vi "TDMS_export_tool.vi"() -> ()   [LabVIEW 2018]
doc: "Tool for exporting TDMS files into CSV format."
uses:
  <vilib>/Utility/miscctls.llb/LVPointTypeDef.ctl
  <vilib>/Platform/TimedLoop/XDataNode/timing_clust.ctl
  <vilib>/Platform/TimedLoop/XDataNode/nitl_modes.ctl
  <vilib>/Platform/TimedLoop/XDataNode/wakeup.ctl
  <vilib>/Utility/sysdir.llb/System Directory Type.ctl
  <vilib>/Platform/TimedLoop/scheduler/LVUserAPI/_suppVIs/Create_1kHz_TSource.vi
  <vilib>/Utility/file.llb/Write Delimited Spreadsheet (string).vi
  <vilib>/platform/TimedLoop/XDataNode/XDataNode.xnode
  <vilib>/Platform/TimedLoop/XDataNode/XDNodeRunTimeDep.lvlib
panel:
  out "error out":errorcluster
  out "Files converted":u32
  out "Settings":bool[](array[boolean])
  out "Data":bool[](array[boolean])
  out "Errors array":string[](array[string])
  in  "Convert":bool
  out "Files to convert":u32
  out "Filelist":path[](array[path])
  in  "Open Folder":bool caption="Open File"
  in  "Stop":bool
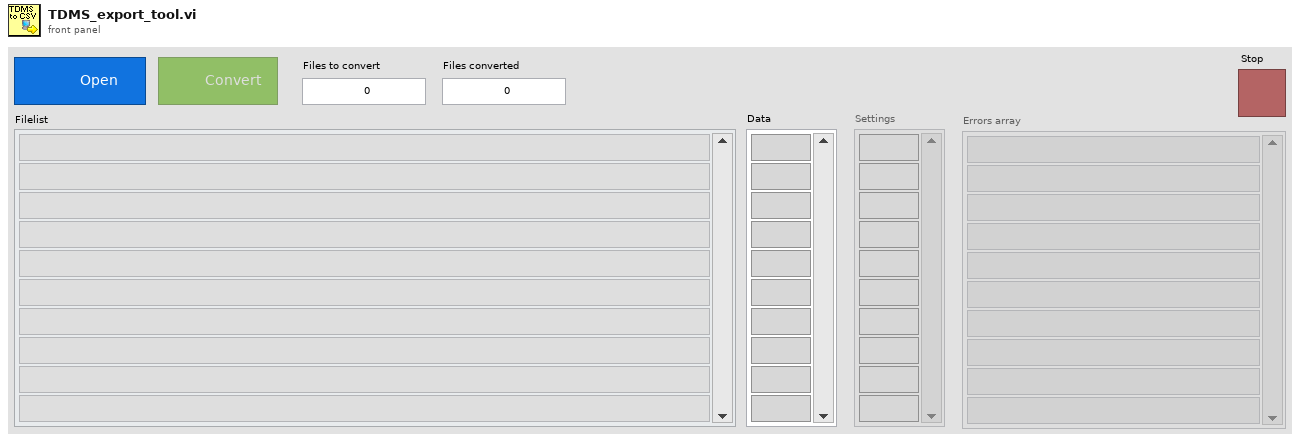
[diagram p1: front panel]
types:
  T1 = enum8{"Enabled", "Disabled", "Disabled and Grayed Out"}
  T2 = typedef "LVPointTypeDef.ctl" = cluster{"Horizontal":i16, "Vertical":i16}
  T3 = typedef "XDNodeRunTimeDep.lvlib/timing_clust.ctl" = cluster{"Expected End [f-1]":u64, "Actual End [f-1]":u64, "Finished Late? [f-1]":bool, "Expected End [i-1]":u64, "Actual End [i-1]":u64, "Finished Late? [i-1]":bool, "Expected Start [i]":u64, "Actual Start [i]":u64, "Expected Start [f]":u64, "Actual Start [f]":u64, "Source Name":string, "Structure Name":string, "Period":i64, "Deadline":i64, "Offset":i64, "Start":i64, "Priority":i32, "Timeout":i32, "Mode":T4, "Wakeup Reason":T5, "Error":errorcluster, "Source Type":string, "Secondary Source Type":string, "Global End Time":u64, "Global Start Time":u64, "Frame Duration":u64, "Iteration Duration":u64, "Assigned CPU":i32, "I/O Scan Engine Mode":u32}
  T4 = typedef "XDNodeRunTimeDep.lvlib/nitl_modes.ctl" = enum32{"No Change", "Process missed periods, maintain original phase", "Discard missed periods, maintain original phase", "Process missed periods, ignore original phase", "Discard missed periods, ignore original phase"}
  T5 = typedef "XDNodeRunTimeDep.lvlib/wakeup.ctl" = enum32{"Normal", "Aborted", "Asynchronous wakeup", "Timing source error", "Timed loop error", "Timeout"}
  T6 = enum32{"invalid app kind", "Development System", "Run Time System", "Student Edition", "Embedded LabVIEW", "Evaluation", "Custom"}
  T7 = typedef "System Directory Type.ctl" = i32
  T8 = cluster{"Raw coordinates data":dbl[][], "Absolute timestamp":string[], "Relative timestamp":string[], "Coordinates and speed":dbl[][], "Current zone and TTLs":u8[][], "Zones preference":string[], "Frame OK":u8[], "Stimulus presets array":cluster{"Event type":u16, "Time, s":sgl, "Stimulus, s":sgl, "Set/Clear":bool, "TTL out":u16, "Stim. has been set":bool}[], "Acquisition settings cluster out":cluster{"Researcher name":string, "N segments MIDFIELD":u8, "N segments BORDER":u8, "Radius, mm CENTER":u16, "Radius, mm MIDFIELD":u16, "Starting angle MIDFIELD":i16, "Starting angle BORDER":i16, "Cage diameter, mm":u16, "Bridge swap":bool, "Bridge V. offset":sgl, "Twisted neck":bool, "Offset H.":sgl, "Name prefix":string, "Stop at":dbl, "\"Stop at\" enabled":bool, "Settings loaded OK":bool}}
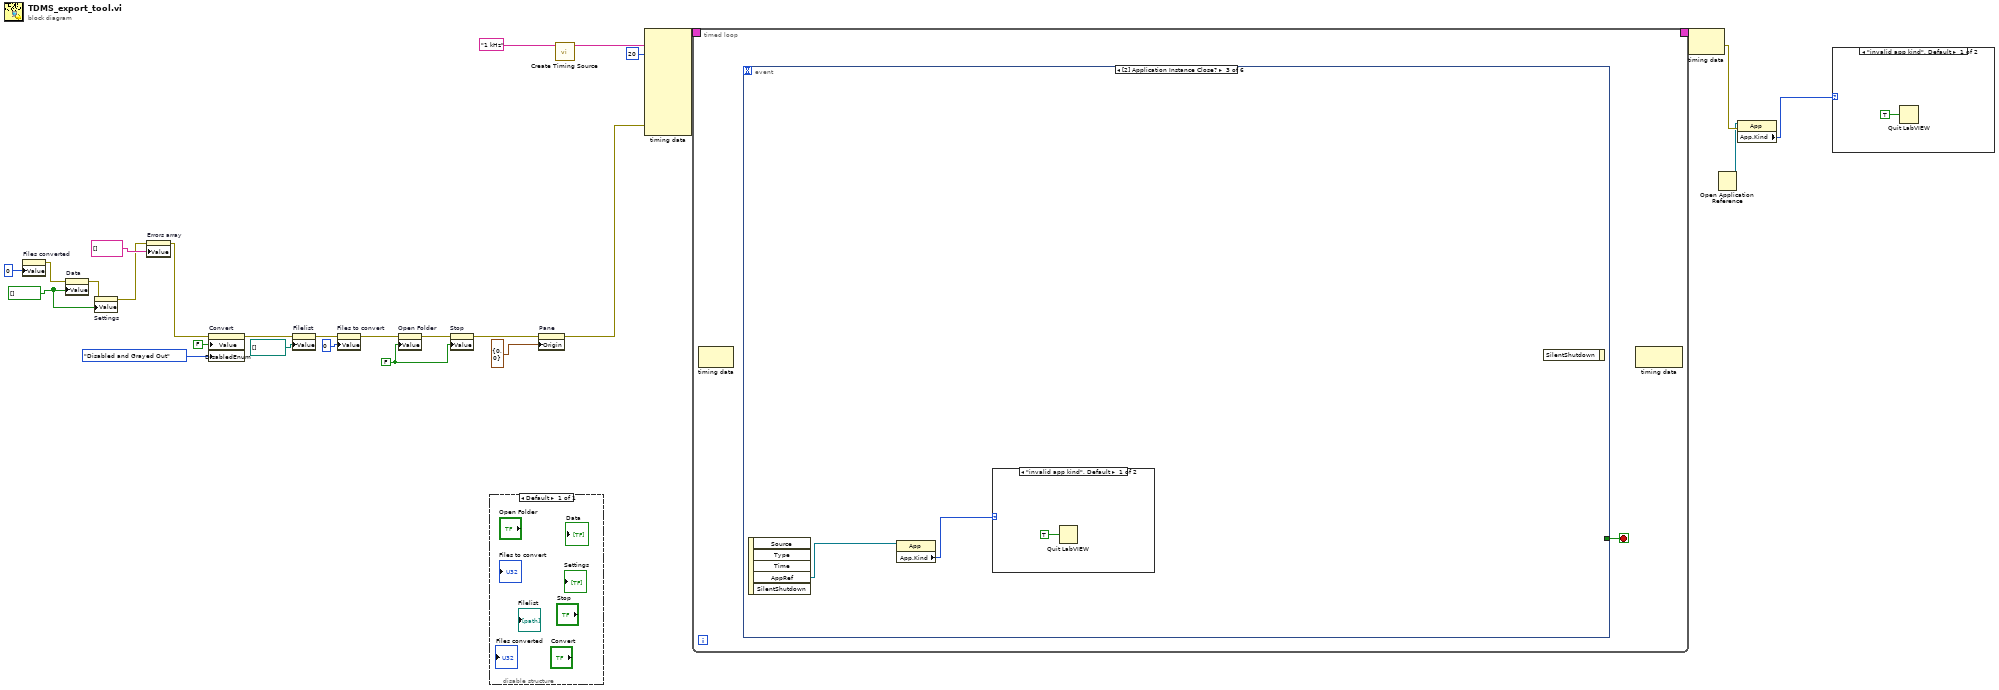
[diagram p0: block diagram]
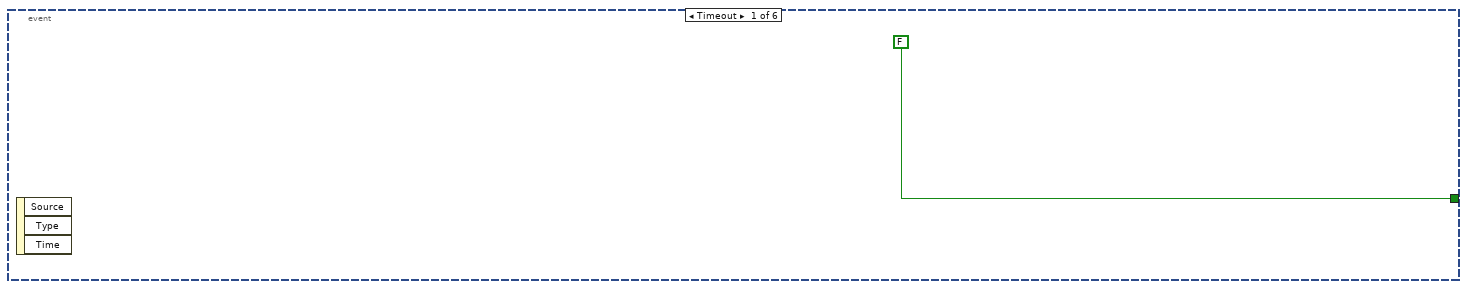
[diagram p3: hidden frame]
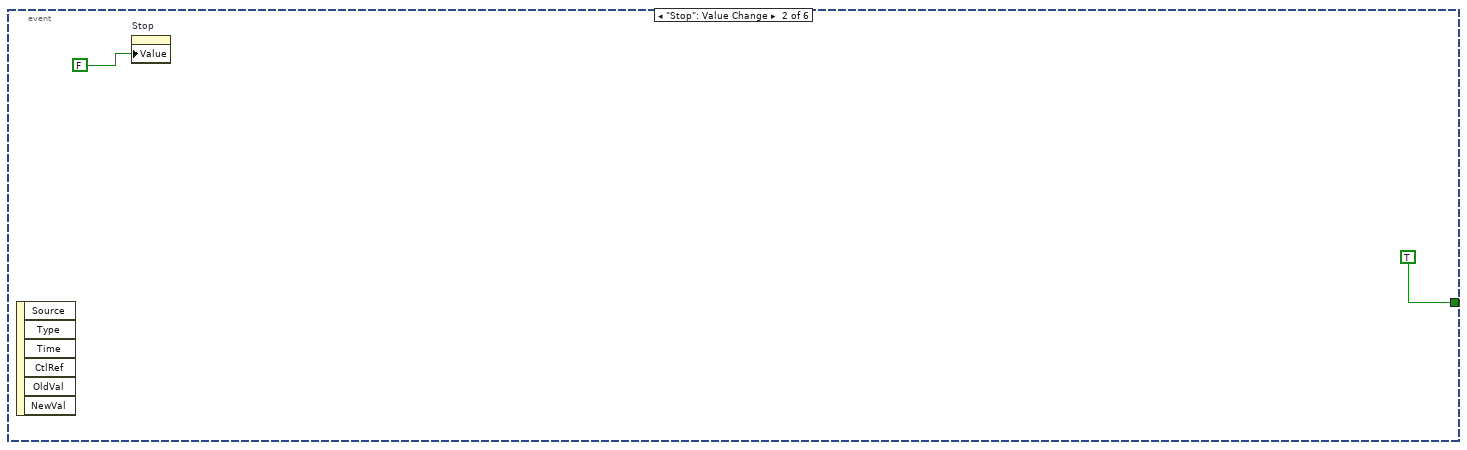
[diagram p4: hidden frame]
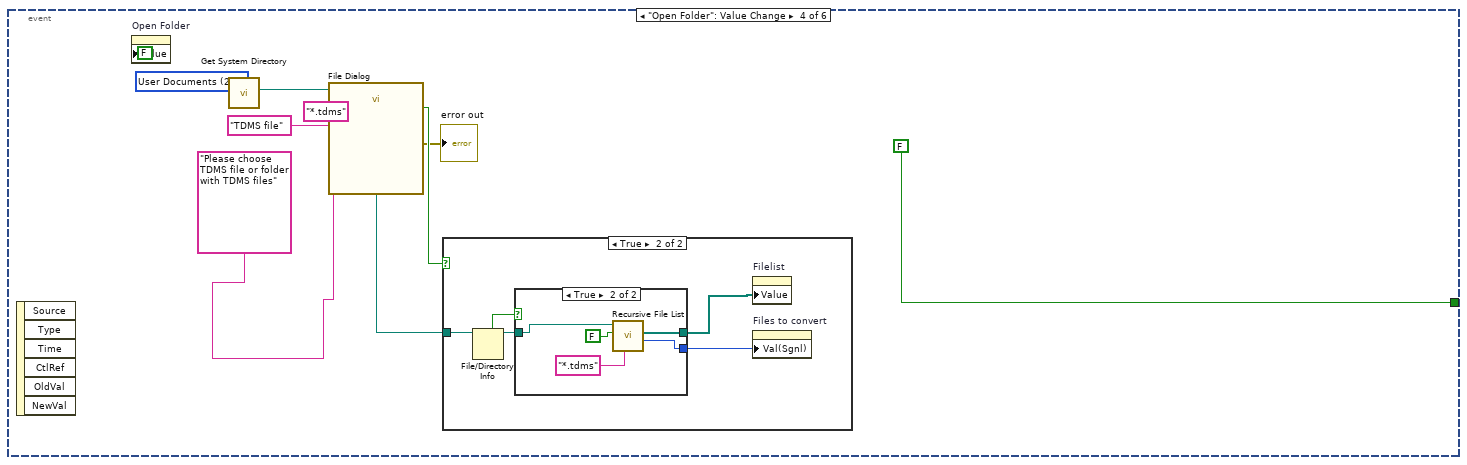
[diagram p6: hidden frame]
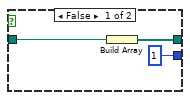
[diagram p8: hidden frame]
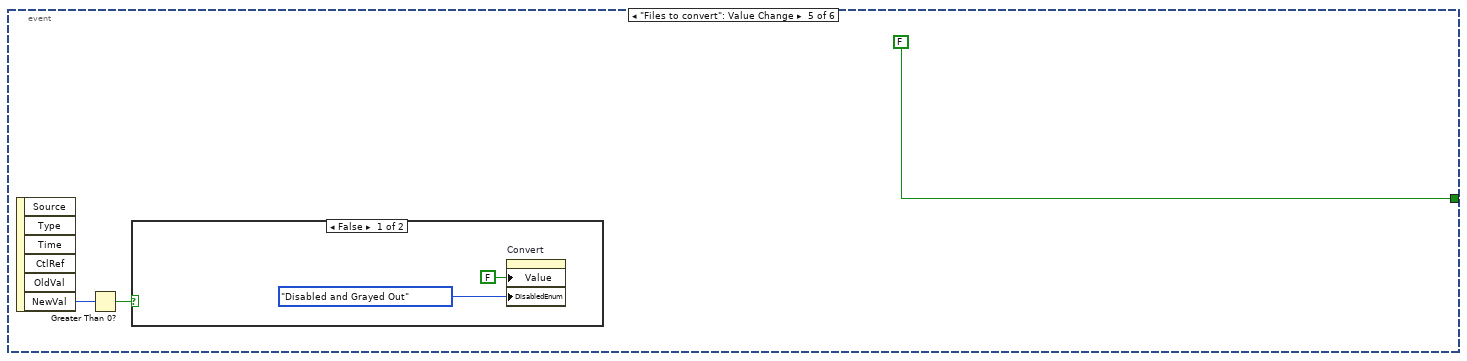
[diagram p9: hidden frame]
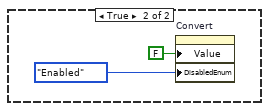
[diagram p10: hidden frame]
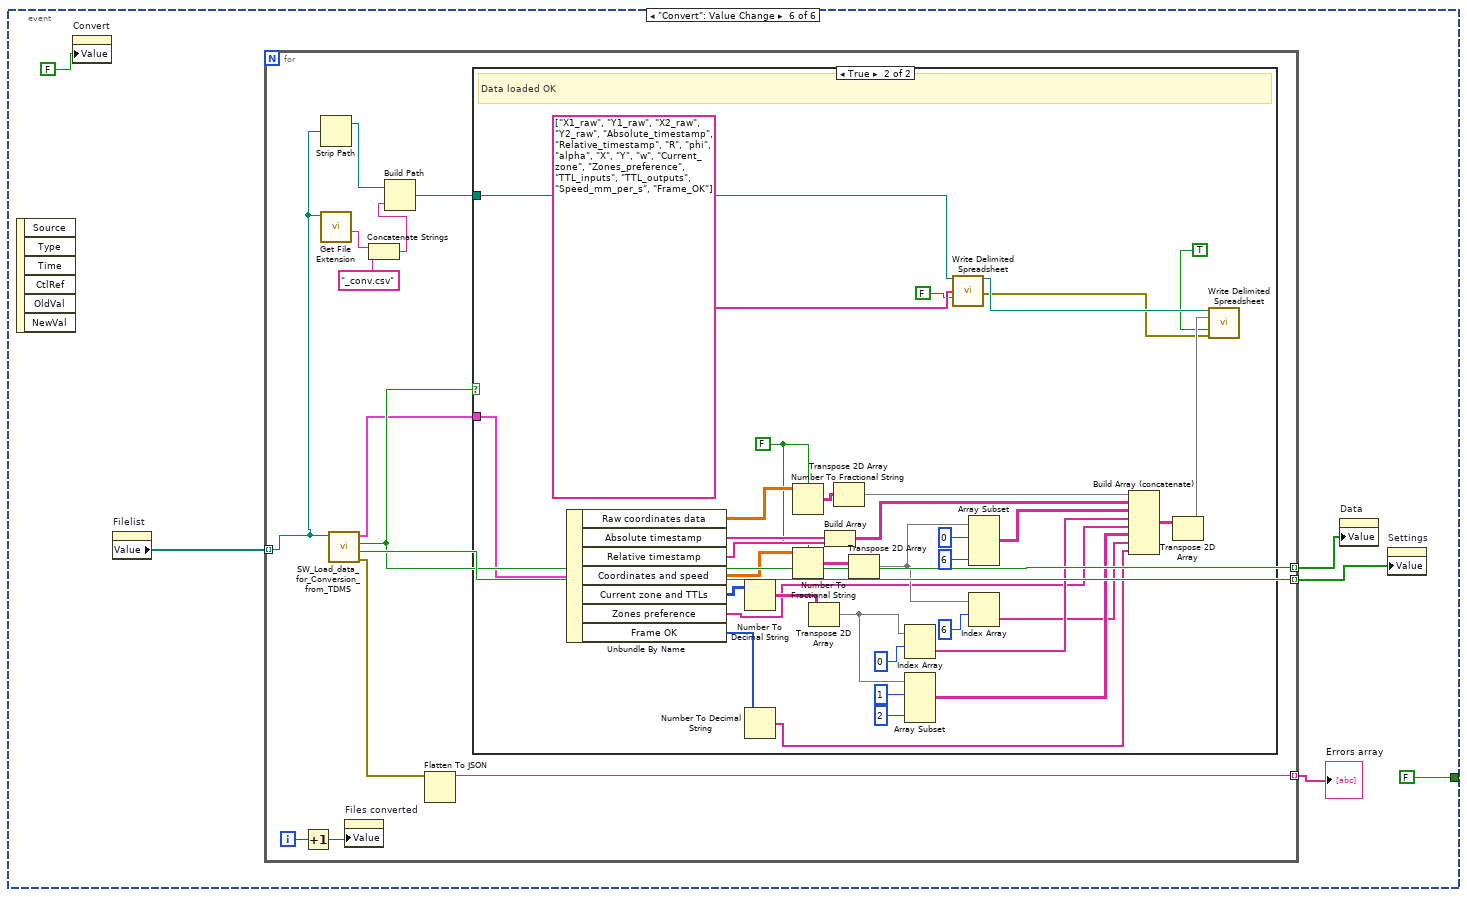
[diagram p11: hidden frame]
diagram:
  w8 = bool[] [] ("Array")
  w18 = FALSE ("Stop")
  n1 = property on="Files converted" class="DigNum (strict)"("Value"=u32 0 ("Files to converted")) -> (error out=w5:errorcluster)  [unwired: 2 in, 1 out]
  n2 = property on="Data" class="Arr"(error in=w5, "Value"=w8) -> (error out=w7:errorcluster)  [unwired: 1 in, 1 out]
  n3 = property on="Settings" class="Arr"(error in=w7, "Value"=w8) -> (error out=w6:errorcluster)  [unwired: 1 in, 1 out]
  n4 = property on="Errors array" class="Arr (strict)"(error in=w6, "Value"=string[] []) -> (error out=w10:errorcluster)  [unwired: 1 in, 1 out]
  n5 = property on="Convert" class="Bool (strict)"(error in=w10, "Value"=FALSE ("Convert"), "DisabledEnum"=T1."Disabled and Grayed Out" ("Disabled")) -> (error out=w13:errorcluster)  [unwired: 1 in, 1 out]
  n6 = property on="Filelist" class="Arr (strict)"(error in=w13, "Value"=path[] [] ("Files to process")) -> (error out=w14:errorcluster)  [unwired: 1 in, 1 out]
  n7 = property on="Files to convert" class="DigNum (strict)"(error in=w14, "Value"=u32 0 ("Number of files")) -> (error out=w17:errorcluster)  [unwired: 1 in, 1 out]
  n8 = property on="Open Folder" class="Bool (strict)"(error in=w17, "Value"=w18) -> (error out=w19:errorcluster)  [unwired: 1 in, 1 out]
  n9 = property on="Stop" class="Bool (strict)"(error in=w19, "Value"=w18) -> (error out=w20:errorcluster)  [unwired: 1 in, 1 out]
  n10 = disable-structure shown="Default" {
    frame Enabled {
    }
  }
  n11 = property on="Pane" class="Pane"(error in=w20, "Origin"=T2 {"Horizontal"=0, "Vertical"=0}) -> (error out=w21:errorcluster)  [unwired: 1 in, 1 out]
  n12 = call-poly <vilib>:"Create Timing Source.vi"("name (in)"="1 kHz") -> ("name (out)"=w24:string)  [unwired: 9 in, 1 out]
  n13 = node-c288(w24, i64 20 ("Period"), w21) -> (w27:T3)  [unwired: 7 in]
  n14 = timed-loop {
    timing: w27 -> [_]
    timing-out: [_] -> w26
    stop <- w28 stop-if-true
    n15 = node-c288() -> ()  [unwired: 1 in, 1 out]
    n16 = event shown="[2] Application Instance Close?" {
      selector: _ -> [_ _ _ _ _ _]
      dyn-events: _ -> [_ _ _ _ _ _]
      timeout: _ -> [_ _ _ _ _ _]
      tunnel: [FALSE TRUE _ FALSE FALSE FALSE] -> w28
      event Timeout {
        n17 = event-data() -> ()  [unwired: 1 in, 3 out]
      }
      event "Stop": Value Change {
        n18 = event-data() -> ()  [unwired: 1 in, 6 out]
        n19 = property on="Stop" class="Bool (strict)"("Value"=FALSE ("Stop")) -> ()  [unwired: 2 in, 2 out]
      }
      event Application Instance Close? {
        n20 = event-data() -> ("AppRef"=w33:refnum<vi>)  [unwired: 1 in, 4 out]
        n21 = property class="App"(reference=w33) -> ("App.Kind"=w32:T6)  [unwired: 1 in, 2 out]
        n22 = case shown="\"invalid app kind\", Default" w32 {
          frame "invalid app kind", Default {
            n23 = Quit LabVIEW(quit? (T)=TRUE) -> ()
          }
          frame "Development System" {
          }
        }
        n24 = event-data() -> ()  [unwired: 2 in, 1 out]
      }
      event "Open Folder": Value Change {
        w40 = T7 2 items=["User Home"=0, "User Desktop"=1, "User Documents"=2, "User Application Data"=3, "User Preferences"=4, "User Temporary"=5, "Public Documents"=6, "Public Application Data"=7, "Public Preferences"=8, "Public Cache"=13, "System Core Libraries"=9, "System Installed Libraries"=10, "Application Files"=11, "Boot Volume Root"=12] ("system directory type")
        n25 = event-data() -> ()  [unwired: 1 in, 6 out]
        n26 = property on="Open Folder" class="Bool (strict)"("Value"=FALSE ("Open Folder")) -> ()  [unwired: 2 in, 2 out]
        n27 = call <vilib>:"Get System Directory.vi"("system directory type"=w40) -> ("system directory"=w39:path)  [unwired: 10 in]
        n28 = call "File Dialog"("start path"=w39, "prompt"="Please choose TDMS file or folder with TDMS files", "pattern (all files)"="*.tdms", "pattern label"="TDMS file") -> ("selected path"=w36:path, "exists"=w37:bool, "error out"=→"error out":errorcluster)  [unwired: 8 in, 1 out]
        n29 = case shown="True" w37 {
          tunnel: w36 -> [_ w49]
          frame False {
          }
          frame True {
            n30 = File/Directory Info(path=w49) -> (path out=w47:path, directory=w48:bool)  [unwired: 1 in, 5 out]
            n31 = case shown="True" w48 {
              tunnel: [w51 w54] -> w45
              tunnel: w47 -> [w52 w57]
              tunnel: [u32 1 ("Number of Files") w53] -> w46
              frame False {
                n32 = Build Array(w52) -> (w51:path[])
              }
              frame True {
                n33 = call <vilib>:"Recursive File List.vi"("pattern"="*.tdms", "Treat LLBs as Folders?"=FALSE, "Folder Path"=w57) -> ("Number of Files"=w53:i32, "All Files in Dir"=w54:path[])  [unwired: 4 in, 3 out]
              }
            }
            n34 = property on="Filelist" class="Arr (strict)"("Value"=w45) -> ()  [unwired: 2 in, 2 out]
            n35 = property on="Files to convert" class="DigNum (strict)"("Val(Sgnl)"=w46) -> ()  [unwired: 2 in, 2 out]
          }
        }
      }
      event "Files to convert": Value Change {
        n36 = event-data() -> ("NewVal"=w59:u32)  [unwired: 1 in, 5 out]
        n37 = Greater Than 0?(x=w59) -> (x > 0?=w58:bool)
        n38 = case shown="False" w58 {
          frame False {
            n39 = property on="Convert" class="Bool (strict)"("Value"=FALSE ("Convert"), "DisabledEnum"=T1."Disabled and Grayed Out" ("Disabled")) -> ()  [unwired: 2 in, 2 out]
          }
          frame True {
            n40 = property on="Convert" class="Bool (strict)"("Value"=FALSE ("Convert"), "DisabledEnum"=T1."Enabled" ("Disabled")) -> ()  [unwired: 2 in, 2 out]
          }
        }
      }
      event "Convert": Value Change {
        n41 = event-data() -> ()  [unwired: 1 in, 6 out]
        n42 = property on="Convert" class="Bool (strict)"("Value"=FALSE ("Convert")) -> ()  [unwired: 2 in, 2 out]
        n43 = property on="Filelist" class="Arr (strict)"() -> ("Value"=w69:path[])  [unwired: 2 in, 2 out]
        n44 = for {
          tunnel: w69 -> [w78] mode=indexing
          tunnel: [w83] -> w67 mode=indexing
          tunnel: [w80] -> w66 mode=indexing
          tunnel: [w81] -> w65 mode=indexing
          i -> [w72]
          n45 = Increment(x=w72) -> (x+1=w71:i32)
          n46 = Strip Path(path=w78) -> (stripped path=w77:path)  [unwired: 1 out]
          n47 = call <vilib>:"Get File Extension.vi"("file"=w78) -> ("filename without extension"=w76:string)  [unwired: 6 in, 4 out]
          n48 = call "SW_Load_data_for_Conversion_from_TDMS.vi"("Path to TDMS file"=w78) -> ("error out"=w82:errorcluster, "Settings loaded OK"=w81:bool, "Data loaded OK"=w80:bool, "Loaded data"=w79:T8)  [unwired: 4 in, 3 out]
          n49 = property on="Files converted" class="DigNum (strict)"("Value"=w71) -> ()  [unwired: 2 in, 2 out]
          n50 = Concatenate Strings(w76, "_conv.csv" ("string")) -> (w74:string)
          n51 = Build Path(base path=w77, name or relative path=w74) -> (appended path=w73:path)
          n52 = Flatten To JSON(anything=w82) -> (JSON string=w83:string)  [unwired: 2 in, 1 out]
          n53 = case shown="True" w80 {
            tunnel: w79 -> [_ w118]
            tunnel: w73 -> [_ w116]
            frame False {
              # "Data is not loaded"
            }
            frame True {
              w103 = FALSE ("use system decimal point (T)")
              # "Data loaded OK"
              n54 = Unbundle By Name(w118) -> ("Raw coordinates data"=w115:dbl[][], "Absolute timestamp"=w113:string[], "Relative timestamp"=w112:string[], "Coordinates and speed"=w110:dbl[][], "Current zone and TTLs"=w107:u8[][], "Zones preference"=w94:string[], "Frame OK"=w105:u8[])
              n55 = Number To Decimal String(number=w107) -> (decimal integer string=w106:string[][])  [unwired: 1 in]
              n56 = Number To Decimal String(number=w105) -> (decimal integer string=w88:string[])  [unwired: 1 in]
              n57 = Number To Fractional String(use system decimal point (T)=w103, number=w115) -> (F-format string=w114:string[][])  [unwired: 2 in]
              n58 = Number To Fractional String(use system decimal point (T)=w103, number=w110) -> (F-format string=w102:string[][])  [unwired: 2 in]
              n59 = Transpose 2D Array(2D array=w106) -> (transposed array=w93:string[][])
              n60 = Build Array(w113, w112) -> (w109:string[][])
              n61 = Transpose 2D Array(2D array=w114) -> (transposed array=w108:string[][])
              n62 = Transpose 2D Array(2D array=w102) -> (transposed array=w100:string[][])
              n63 = Index Array(array=w93, index (row)=0) -> (element=w95:string[])  [unwired: 1 in]
              n64 = Array Subset(array=w93, index (row)=1 ("index"), length (row)=2 ("length")) -> (w90:string[][])  [unwired: 2 in]
              n65 = call-poly <vilib>:"Write Delimited Spreadsheet.vi"("file path (dialog if empty)"=w116, "1D data"=string[] ["X1_raw", "Y1_raw", "X2_raw", "Y2_raw", "Absolute_timestamp", "Relative_timestamp", "R", "phi", "alpha", "X", "Y", "w", "Current_zone", "Zones_preference", "TTL_inputs", "TTL_outputs", "Speed_mm_per_s", "Frame_OK"] ("appended array"), "append to file? (new file:F)"=FALSE) -> ("new file path (Not A Path if cancelled)"=w86:path, "error out"=w84:errorcluster)  [unwired: 11 in]
              n66 = Array Subset(array=w100, index (row)=0 ("index"), length (row)=6 ("length")) -> (w97:string[][])  [unwired: 2 in]
              n67 = Index Array(array=w100, index (row)=6) -> (element=w89:string[])  [unwired: 1 in]
              n68 = Build Array (concatenate)(w108, w109, w97, w95, w94, w90, w89, w88) -> (w111:string[][])
              n69 = Transpose 2D Array(2D array=w111) -> (transposed array=w104:string[][])
              n70 = call-poly <vilib>:"Write Delimited Spreadsheet.vi"("file path (dialog if empty)"=w86, "2D data"=w104, "append to file? (new file:F)"=TRUE, "error in (no error)"=w84) -> ()  [unwired: 10 in, 2 out]
            }
          }
        }
        "Errors array" <- w67
        n71 = property on="Data" class="Arr"("Value"=w66) -> ()  [unwired: 2 in, 2 out]
        n72 = property on="Settings" class="Arr"("Value"=w65) -> ()  [unwired: 2 in, 2 out]
      }
    }
    n73 = node-c288() -> ()  [unwired: 1 in, 1 out]
  }
  n74 = node-c288(w26) -> (w2:errorcluster)
  n75 = Open Application Reference() -> (3:w1:refnum<vi>)  [unwired: 4 in, 1 out]
  n76 = property class="App"(reference=w1, error in=w2) -> ("App.Kind"=w3:T6)  [unwired: 2 out]
  n77 = case shown="\"invalid app kind\", Default" w3 {
    frame "invalid app kind", Default {
      n78 = Quit LabVIEW(quit? (T)=TRUE) -> ()
    }
    frame "Development System" {
    }
  }
